vi "Close TLCamera.vi"(8 "error in (no error)":errorcluster, 11 "TLCamera reference":refnum<k24>) -> (0 "error out":errorcluster)   [LabVIEW 2022 SP3]
uses:
  I:/.shortcut-targets-by-id/1riZacJd_1_jmKfGgrjDuP7KcecvMS3i2/Xiao research group/Programs/XYZRecorrection/Scientific Camera Interfaces/SDK/DotNet Toolkit/dlls/Managed_64_lib/Thorlabs.TSI.TLCamera.dll
  SDK/DotNet Toolkit/dlls/Managed_64_lib/Thorlabs.TSI.TLCamera.dll
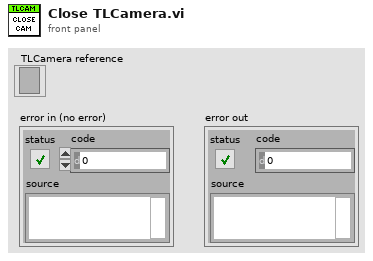
[diagram p1: front panel]
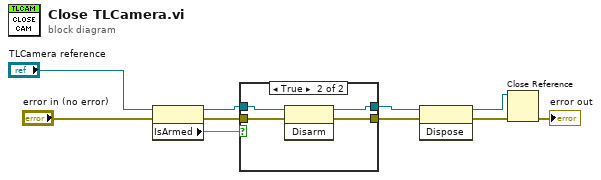
[diagram p0: block diagram]
diagram:
  n1 = property(reference="TLCamera reference", error in="error in (no error)") -> (reference out=w3:refnum<k24>, error out=w5:errorcluster, "IsArmed"=w2)
  n2 = case shown="True" w2 {
    tunnel: w3 -> [w12 w16]
    tunnel: w5 -> [w11 w15]
    tunnel: [w12 w14] -> w6
    tunnel: [w11 w13] -> w7
    frame False {
    }
    frame True {
      n3 = invoke method="Disarm"(reference=w16, error in=w15) -> (reference out=w14:refnum<k24>, error out=w13:errorcluster)  [unwired: 1 in, 1 out]
    }
  }
  n4 = invoke method="Dispose"(reference=w6, error in=w7) -> (reference out=w9:refnum<k24>, error out=w8:errorcluster)  [unwired: 1 in, 1 out]
  n5 = Close Reference(reference=w9, error in (no error)=w8) -> (error out=→"error out":errorcluster)
